vi "Close Child.vi"(8 "error in (no error)":errorcluster, 11 "Websocket Server in":refnum<class "Websocket Server.lvclass">) -> (0 "error out":errorcluster, 3 "Websocket Server out":refnum<class "Websocket Server.lvclass">)   [LabVIEW 2020, in "Stream-Websocket.lvlib" / "Websocket Server.lvclass"]
uses:
  Websocket Server.lvclass
  Websocket Server.lvclass/Websocket Server.ctl
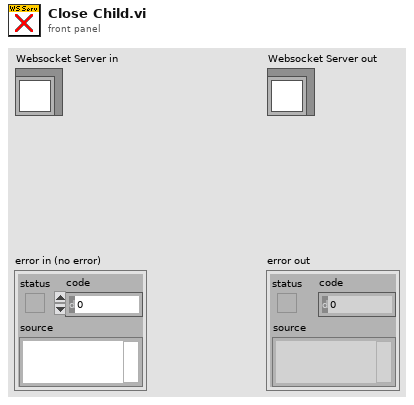
[diagram p1: front panel]
types:
  T1 = typedef "Stream-Websocket.lvlib/Websocket Server.lvclass/Ref Data.ctl" = cluster{"Listener":refnum<k5>, "Clients":refnum<class "Websocket Client.lvclass">[], "Server Loop":bool}
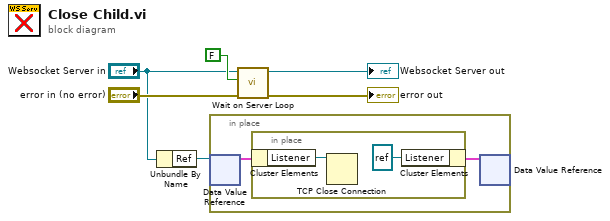
[diagram p0: block diagram]
diagram:
  n1 = Unbundle By Name("Websocket Server in") -> ("Ref"=w2:refnum<data-value>)
  n2 = in-place {
    n3 = in-place-dvr #1(w2) -> (w8:T1)  [unwired: 1 out]
    n4 = in-place {
      n5 = in-place-cluster #2(w8) -> ("Listener"=w10:refnum<k5>)
      n6 = TCP Close Connection(connection ID=w10) -> ()  [unwired: 2 in, 2 out]
      n7 = in-place-cluster #2("Listener"=refnum<k5> refnum) -> (w7:T1)
    }
    n8 = in-place-dvr #1(w7) -> ()  [unwired: 2 out]
  }
  n9 = call "Wait on Server Loop.vi"("error in (no error)"="error in (no error)", "Value"=FALSE, "Websocket Server in"="Websocket Server in") -> ("error out"=→"error out":errorcluster, "Websocket Server out"=→"Websocket Server out":refnum<class "Websocket Server.lvclass">)  [unwired: 7 in]
